vi "GetMetadataVariable.vi"(9 "Default Value":string, 10 "Variable name":string, 11 "input string":string) -> (1 "remaining string":string, 2 "Found Variable?":bool, 3 "Variable Value":string)   [LabVIEW 2015]
uses:
  <vilib>/regexp/Match Regular Expression.xnode
panel:
  out "after substring":string
  out "before substring":string
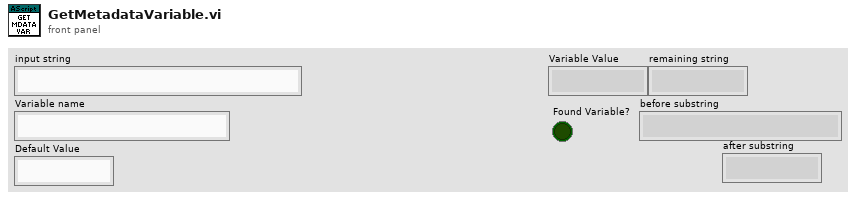
[diagram p1: front panel]
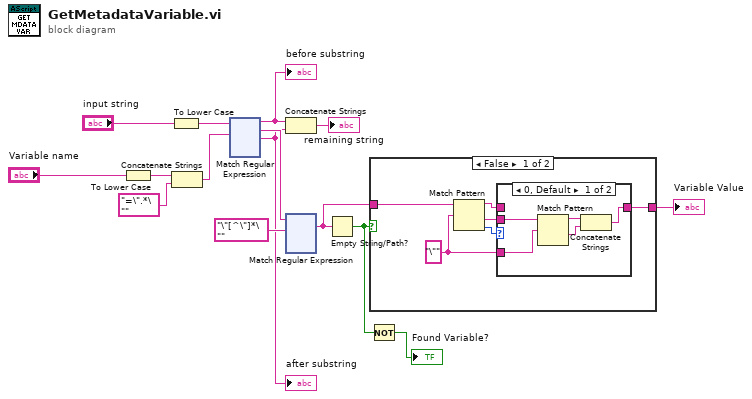
[diagram p0: block diagram]
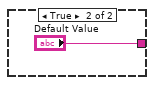
[diagram p3: hidden frame]
diagram:
  n1 = To Lower Case(string="Variable name") -> (all lower case string=w12:string)
  n2 = To Lower Case(string="input string") -> (all lower case string=w11:string)
  n3 = Concatenate Strings(w12, "=\".*\"" ("expression")) -> (w10:string)
  n4 = xnode "Match Regular Expression"("input string"=w11, "regular expression"=w10) -> ("before match"=w3:string, "whole match"=w9:string, "after match"=w2:string)  [unwired: 4 in, 2 out]
  "before substring" <- w3
  "after substring" <- w2
  n5 = Concatenate Strings(w3, w2) -> (→"remaining string":string)
  n6 = xnode "Match Regular Expression"("input string"=w9, "regular expression"="\"[^\"]*\"") -> ("whole match"=w6:string)  [unwired: 4 in, 4 out]
  n7 = Empty String/Path?(string/path=w6) -> (empty?=w5:bool)
  n8 = Not(x=w5) -> (.not. x?=→"Found Variable?":bool)
  n9 = case shown="False" w5 {
    tunnel: [w17 "Default Value"] -> w7
    tunnel: w6 -> [w16 _]
    frame False {
      w18 = "\"" ("replace string (\"\")")
      n10 = Match Pattern(string=w16, regular expression=w18) -> (before substring=w20:string, after substring=w19:string, offset past match=w21:i32)  [unwired: 2 out]
      n11 = case shown="0, Default" w21 {
        tunnel: w18 -> [w24 _]
        tunnel: w20 -> [_ w27]
        tunnel: [w23 w27] -> w17
        tunnel: w19 -> [w26 _]
        frame 0, Default {
          n12 = Match Pattern(string=w26, regular expression=w24) -> (before substring=w25:string, after substring=w22:string)  [unwired: 3 out]
          n13 = Concatenate Strings(w25, w22) -> (w23:string)
        }
        frame -1 {
        }
      }
    }
    frame True {
    }
  }
  "Variable Value" <- w7
